vi "Pressure Sensor-Dual.vi"() -> ()   [LabVIEW 2009]
uses:
  <vilib>/NXT/Block Support/NXT_InputPort.ctl
  <vilib>/NXT/Subs/LVHSConnector.ctl
  <vilib>/NXT/Dual Mode Library/Display/drawNumber.vi
  <vilib>/NXT/Dual Mode Library/Display/drawText.vi
  mindsensors.com LVEE Toolkit/Dual/Pressure Sensor-DM.vi
panel:
  out "NXT dup":T1
  in  "NXT":T1={"error"={"status"=FALSE, "code"=0, "source"=""}, "address"="", "NXT #"=-1, "Show Error"=TRUE}
  in  "stop":bool
  out "Pressure Guage (psi)":u8(slide)=5 scale=0.0..50.0
  in  "Input":T2 items=["Port 1", "Port 2", "Port 3", "Port 4"]
  out "Pressure (psi)":i16=40
  # "mindsensors.com\nCopyright (c) 2009 by mindsensors.com\nEmail: info (<at>) mindsensors (<dot>) com\n\nThis program is free software. You can redistribute it and/or modify\nit under the terms of the GNU General Public License as published by\nthe Free Software Foundation; version 3 of the License.\nRead the license at: http://www.gnu.org/licenses/gpl.txt"
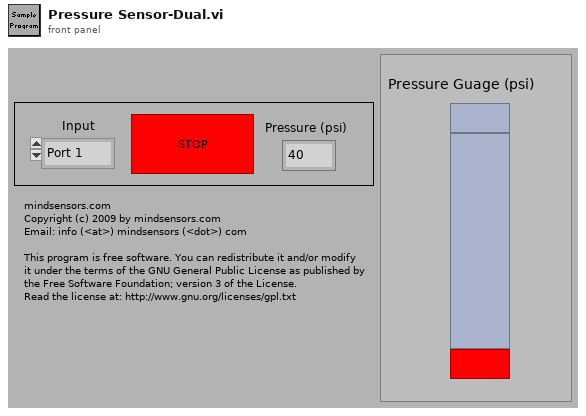
[diagram p1: front panel]
types:
  T1 = typedef "LVHSConnector.ctl" = cluster{"error":errorcluster, "address":string, "NXT #":i32, "Show Error":bool}
  T2 = typedef "NXT_InputPort.ctl" = u8
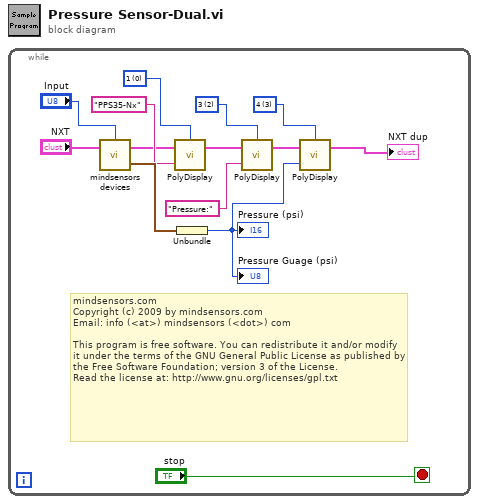
[diagram p0: block diagram]
diagram:
  n1 = while {
    stop <- "stop" stop-if-true
    w7 = i16 3 items=["1", "2", "3", "4", "5", "6", "7", "8"] ("Line")
    w9 = i16 2 items=["1", "2", "3", "4", "5", "6", "7", "8"] ("Line")
    w11 = i16 0 items=["1", "2", "3", "4", "5", "6", "7", "8"] ("Line")
    # "mindsensors.com\nCopyright (c) 2009 by mindsensors.com\nEmail: info (<at>) mindsensors (<dot>) com\n\nThis program is free software. You can redistribute it and/or modify\nit under the terms of the GNU General Public License as published by\nthe Free Software Foundation; version 3 of the License.\nRead the license at: http://www.gnu.org/licenses/gpl.txt"
    n2 = call-poly "mindsensors devices.vi"("NXT"="NXT", "Input Port"="Input") -> ("Pressure (psi)"=w12:cluster{u16}, "NXT dup"=w3:T1)  [unwired: 1 in]
    n3 = call-poly <vilib>:"PolyDisplay.vi"("Text"="PPS35-Nx", "NXT"=w3, "Line"=w11) -> ("NXT"=w4:T1)  [unwired: 1 in]
    n4 = Unbundle(w12) -> (w6:u16)
    "Pressure (psi)" <- w6
    "Pressure Guage (psi)" <- w6
    n5 = call-poly <vilib>:"PolyDisplay.vi"("Text"="Pressure:", "NXT"=w4, "Line"=w9) -> ("NXT"=w5:T1)  [unwired: 1 in]
    n6 = call-poly <vilib>:"PolyDisplay.vi"("number"=w6, "NXT"=w5, "Line"=w7) -> ("NXT"=→"NXT dup":T1)  [unwired: 1 in]
  }
